vi "GetArrayElement.vi"(8 "error in (no error)":errorcluster, 10 "Desired element":dbl=2.5 format="%#_13g", 11 "Array":dbl[](array[numeric])) -> (0 "error out":errorcluster, 2 "New index":i32)   [LabVIEW 2016]
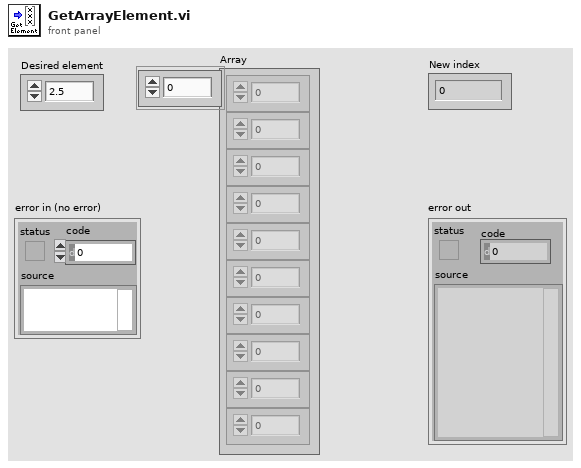
[diagram p1: front panel]
types:
  T1 = enum16{"Left Button", "Center Button", "Right Button", "Window Close"}
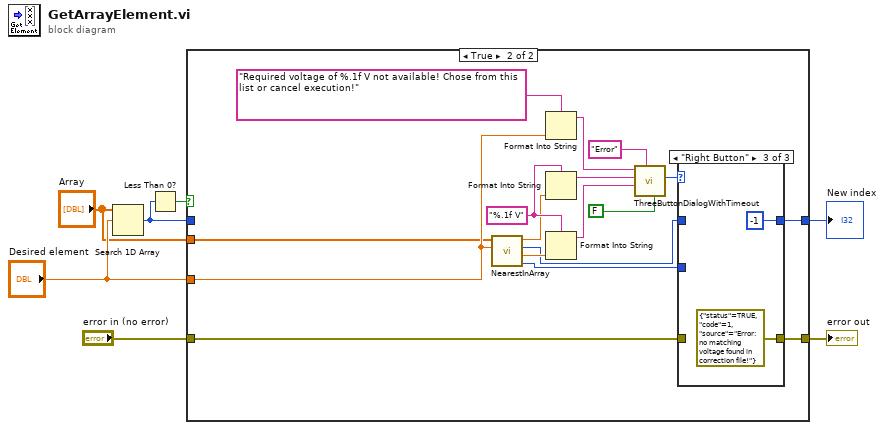
[diagram p0: block diagram]
diagram:
  n1 = Search 1D Array(1D array="Array", element="Desired element") -> (index of element=w5:i32)  [unwired: 1 in]
  n2 = Less Than 0?(x=w5) -> (x < 0?=w7:bool)
  n3 = case shown="True" w7 {
    tunnel: w5 -> [w9 _]
    tunnel: [w9 w18] -> w6
    tunnel: "Array" -> [_ w23]
    tunnel: "Desired element" -> [_ w24]
    tunnel: "error in (no error)" -> [w8 w17]
    tunnel: [w8 w16] -> w1
    frame False {
    }
    frame True {
      w25 = "%.1f V" ("format string")
      n4 = call "NearestInArray.vi"("desired element"=w24, "1D Array"=w23) -> ("2nd closest index"=w20:i32, "2nd closest element"=w21:dbl, "closest index"=w19:i32, "closest element"=w22:dbl)  [unwired: 6 in]
      n5 = Format Into String(format string="Required voltage of %.1f V not available! Chose from this list or cancel execution!" ("Window Title (\"\")"), w24) -> (resulting string=w14:string)  [unwired: 2 in, 1 out]
      n6 = Format Into String(format string=w25, w22) -> (resulting string=w13:string)  [unwired: 2 in, 1 out]
      n7 = Format Into String(format string=w25, w21) -> (resulting string=w12:string)  [unwired: 2 in, 1 out]
      n8 = call "ThreeButtonDialogWithTimeout.vi"("Allow user to close window? (TRUE)"=FALSE, "Window Title (\"\")"="Error" ("Window Title (\"\")"), "Center Button Text (\"No\")"=w12, "Default Button Text (\"Yes\")"=w13, "message"=w14) -> ("Which Button?"=w10:T1)  [unwired: 6 in]
      n9 = case shown="\"Right Button\"" w10 {
        tunnel: w19 -> [w28 _ _]
        tunnel: w20 -> [_ w30 _]
        tunnel: [w28 w30 -1] -> w18
        tunnel: w17 -> [w27 w29 _]
        tunnel: [w27 w29 errorcluster {"status"=TRUE, "code"=1, "source"="Error: no matching voltage found in correction file!"} ("error constant")] -> w16
        frame "Left Button", Default {
        }
        frame "Center Button" {
        }
        frame "Right Button" {
        }
      }
    }
  }
  "New index" <- w6
  "error out" <- w1
